vi "Identity ID.vi"(11 "TaskIdentity in":refnum<class "TaskIdentity.lvclass">) -> (2 "ID":string)   [LabVIEW 2020, in "Volatus.lvlib" / "TaskIdentity.lvclass"]
uses:
  TaskIdentity.lvclass
  TaskIdentity.lvclass/TaskIdentity.ctl
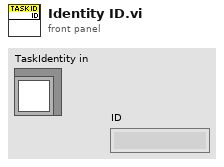
[diagram p1: front panel]
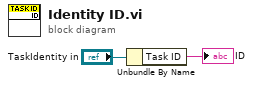
[diagram p0: block diagram]
diagram:
  n1 = Unbundle By Name("TaskIdentity in") -> ("Task ID"=→"ID":string)
